vi "Exercise Cluster.vi"() -> ()   [LabVIEW 2015]
panel:
  out "array of clusters 2":cluster{"String":string, "String":string}[](array[cluster])
  in  "Array 2":string[](array[string])
  in  "Array":string[](array[string])
  out "array of clusters":T1(array[cluster])
  in  "Cluster 4":T2
  in  "Cluster 3":T2
  in  "Cluster 2":T2
  out "output cluster 2":T3
  in  "Boolean 2":bool
  in  "Boolean":bool
  out "dt":dbl
  out "t0":timestamp
  out "Y":dbl[](array[numeric])
  in  "Waveform":waveform(dbl)
  out "output cluster":T4
  in  "Cluster":T5
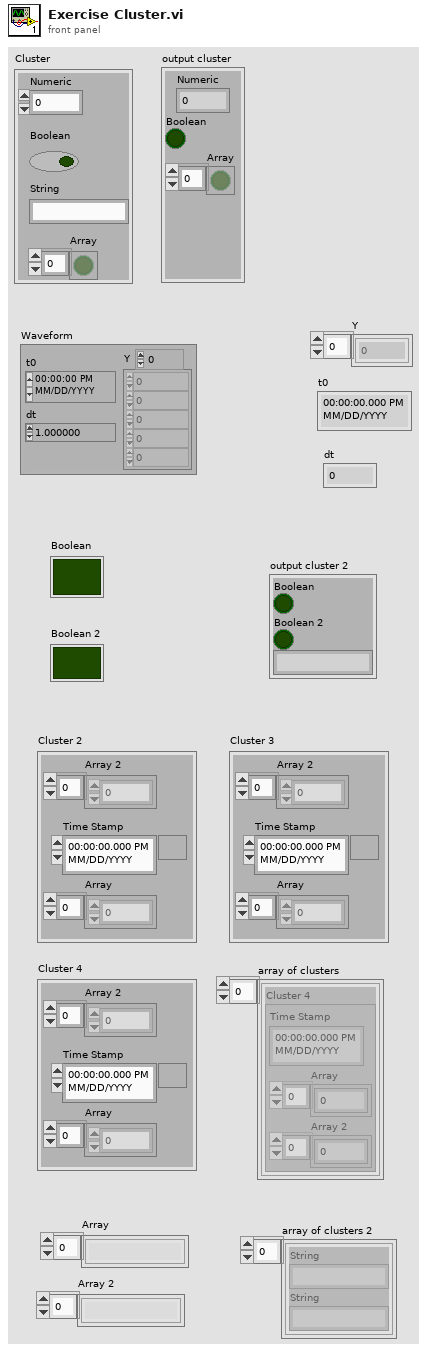
[diagram p1: front panel]
types:
  T1 = cluster{"Cluster 4":cluster{"Time Stamp":timestamp, "Array":dbl[], "Array 2":dbl[]}}[]
  T2 = cluster{"Time Stamp":timestamp, "Array":dbl[], "Array 2":dbl[]}
  T3 = cluster{"Boolean":bool, "Boolean 2":bool, string}
  T4 = cluster{"Numeric":dbl, "Boolean":bool, "Array":bool[]}
  T5 = cluster{"Numeric":dbl, "Boolean":bool, "String":string, "Array":bool[]}
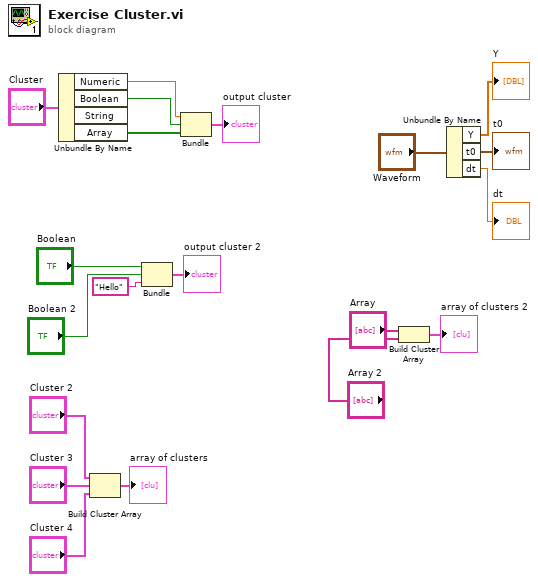
[diagram p0: block diagram]
diagram:
  n1 = Unbundle By Name "Unbundle By Name"("Cluster") -> ("Numeric"=w19:dbl, "Boolean"=w18:bool, "Array"=w17:bool[])  [unwired: 1 out]
  n2 = Build Cluster Array("Cluster 2", "Cluster 3", "Cluster 4") -> (→"array of clusters":T1)
  n3 = Bundle("Boolean"="Boolean", "Boolean 2"="Boolean 2", "Hello") -> (→"output cluster 2":T3)  [unwired: 1 in]
  n4 = Bundle("Numeric"=w19, "Boolean"=w18, "Array"=w17) -> (→"output cluster":T4)  [unwired: 1 in]
  n5 = Build Cluster Array("Array", "Array 2") -> (→"array of clusters 2":cluster{"String":string, "String":string}[])
  n6 = Unbundle By Name("Waveform") -> ("Y"=→"Y":dbl[], "t0"=→"t0":timestamp, "dt"=→"dt":dbl)
